vi "Ideal Center V.4.0.vi"() -> (1 "Center+1":dbl, 2 "Ideal Center":dbl, 3 "Center-1":dbl)   [LabVIEW 2016]
uses:
  Robot Global Data V.5.0.vi
panel:
  # "sets the  ideal x value the target would be at based on distance travelled"
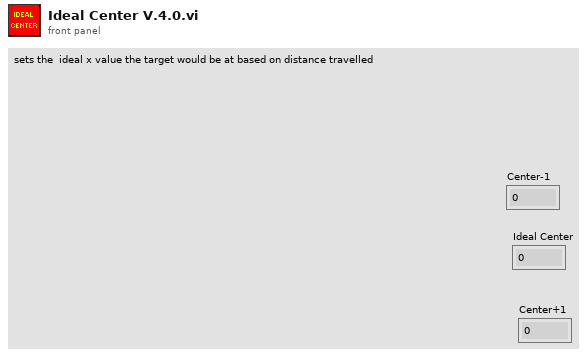
[diagram p1: front panel]
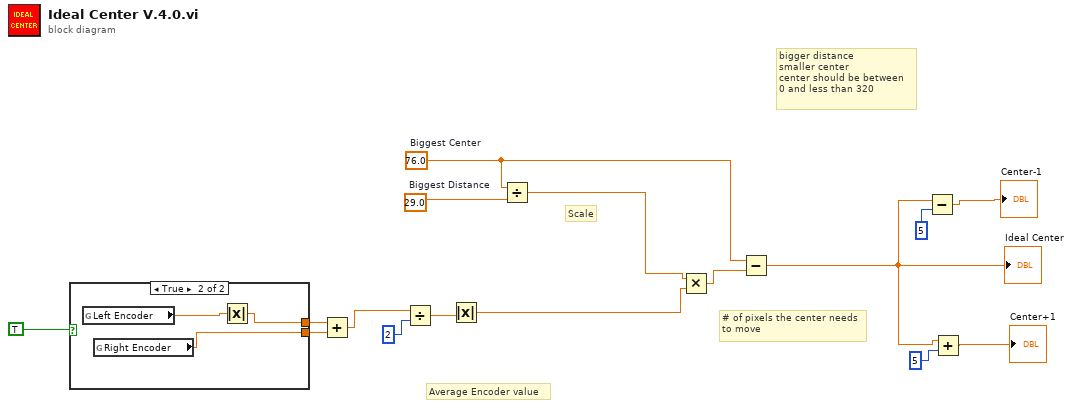
[diagram p0: block diagram]
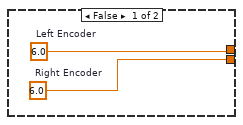
[diagram p2: hidden frame]
diagram:
  w10 = 29.0  # Biggest Distance
  w8 = 76.0  # Biggest Center
  # "# of pixels the center needs\nto move"
  # "Scale"
  # "Average Encoder value"
  # "bigger distance\nsmaller center\ncenter should be between\n0 and less than 320"
  n1 = case shown="True" TRUE {
    tunnel: [w17 w19] -> w15
    tunnel: [w18 w21] -> w13
    frame False {
      w18 = 6.0  # Right Encoder
      w17 = 6.0  # Left Encoder
    }
    frame True {
      n2 = global read "Robot Global Data V.5.0.vi" "Left Encoder"() -> (w20:dbl)
      n3 = global read "Robot Global Data V.5.0.vi" "Right Encoder"() -> (w21:dbl)
      n4 = Absolute Value(x=w20) -> (abs(x)=w19:dbl)
    }
  }
  n5 = Add(x=w15, y=w13) -> (x+y=w14:dbl)
  n6 = Divide(x=w14, y=2) -> (x/y=w7:dbl)
  n7 = Absolute Value(x=w7) -> (abs(x)=w6:dbl)
  n8 = Divide(x=w8, y=w10) -> (x/y=w9:dbl)
  n9 = Multiply(x=w9, y=w6) -> (x*y=w11:dbl)
  n10 = Subtract(x=w8, y=w11) -> (x-y=w4:dbl)
  "Ideal Center" <- w4
  n11 = Subtract(x=w4, y=5) -> (x-y=→"Center-1":dbl)
  n12 = Add(x=w4, y=5) -> (x+y=→"Center+1":dbl)
